vi "test_Timestamp Channel.vi"(8 "error in (no error)":errorcluster, 11 "TestCase in":refnum<class "Instrument Addon Common System Tests.lvclass">) -> (0 "error out":errorcluster, 3 "TestCase out":refnum<class "Instrument Addon Common System Tests.lvclass">)   [LabVIEW 2019, in "Instrument Addon Common System Tests.lvclass"]
uses:
  Instrument Addon Common System Tests.lvclass
  C:/Program Files (x86)/National Instruments/LabVIEW 2019/vi.lib/NI/VeriStand Custom Device Testing Tools/VeriStandTestCase/VeriStandTestCase.lvclass
  8f14a969-7c39-4f15-840b-a7ce507a422e.vi
  <vilib>/NI VeriStand/Execution/Workspace/NI VeriStand - Get Single Channel Value.vi
  <vilib>/NI VeriStand/Execution/Workspace/NI VeriStand - Set Single Channel Value.vi
  <vilib>/addons/_JKI Toolkits/VI Tester/TestCase.llb/TestCase.lvclass
  <vilib>/NI VeriStand/Execution/Workspace/NI_VS Workspace ExecutionAPI.lvlib
  C:/Program Files (x86)/National Instruments/LabVIEW 2019/vi.lib/addons/_JKI Toolkits/VI Tester/TestCase.llb/TestCase.lvclass
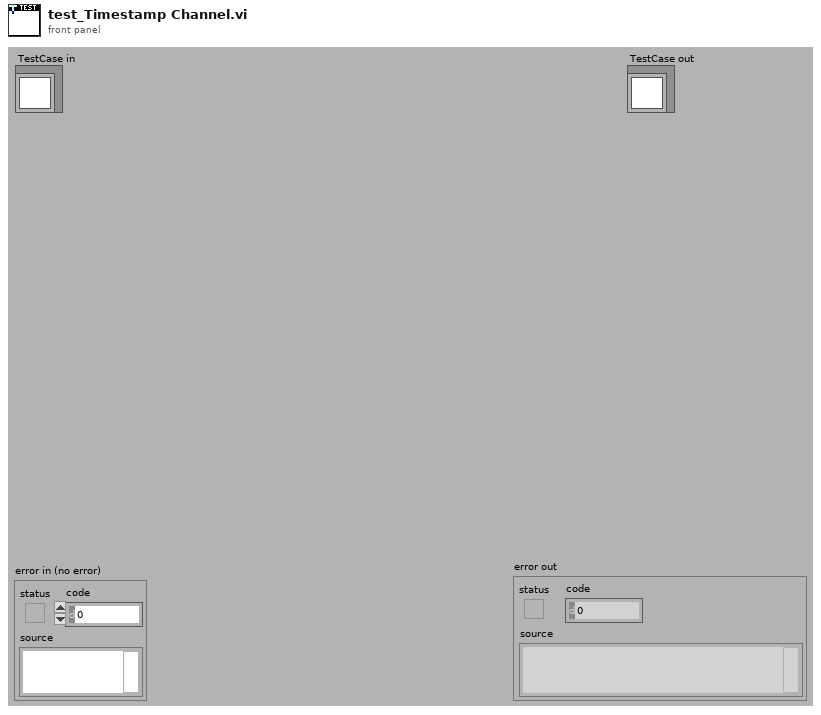
[diagram p1: front panel]
types:
  T1 = typedef "NI_VS Workspace ExecutionAPI.lvlib/WorkspaceAPI.ctl" = refnum<k24>
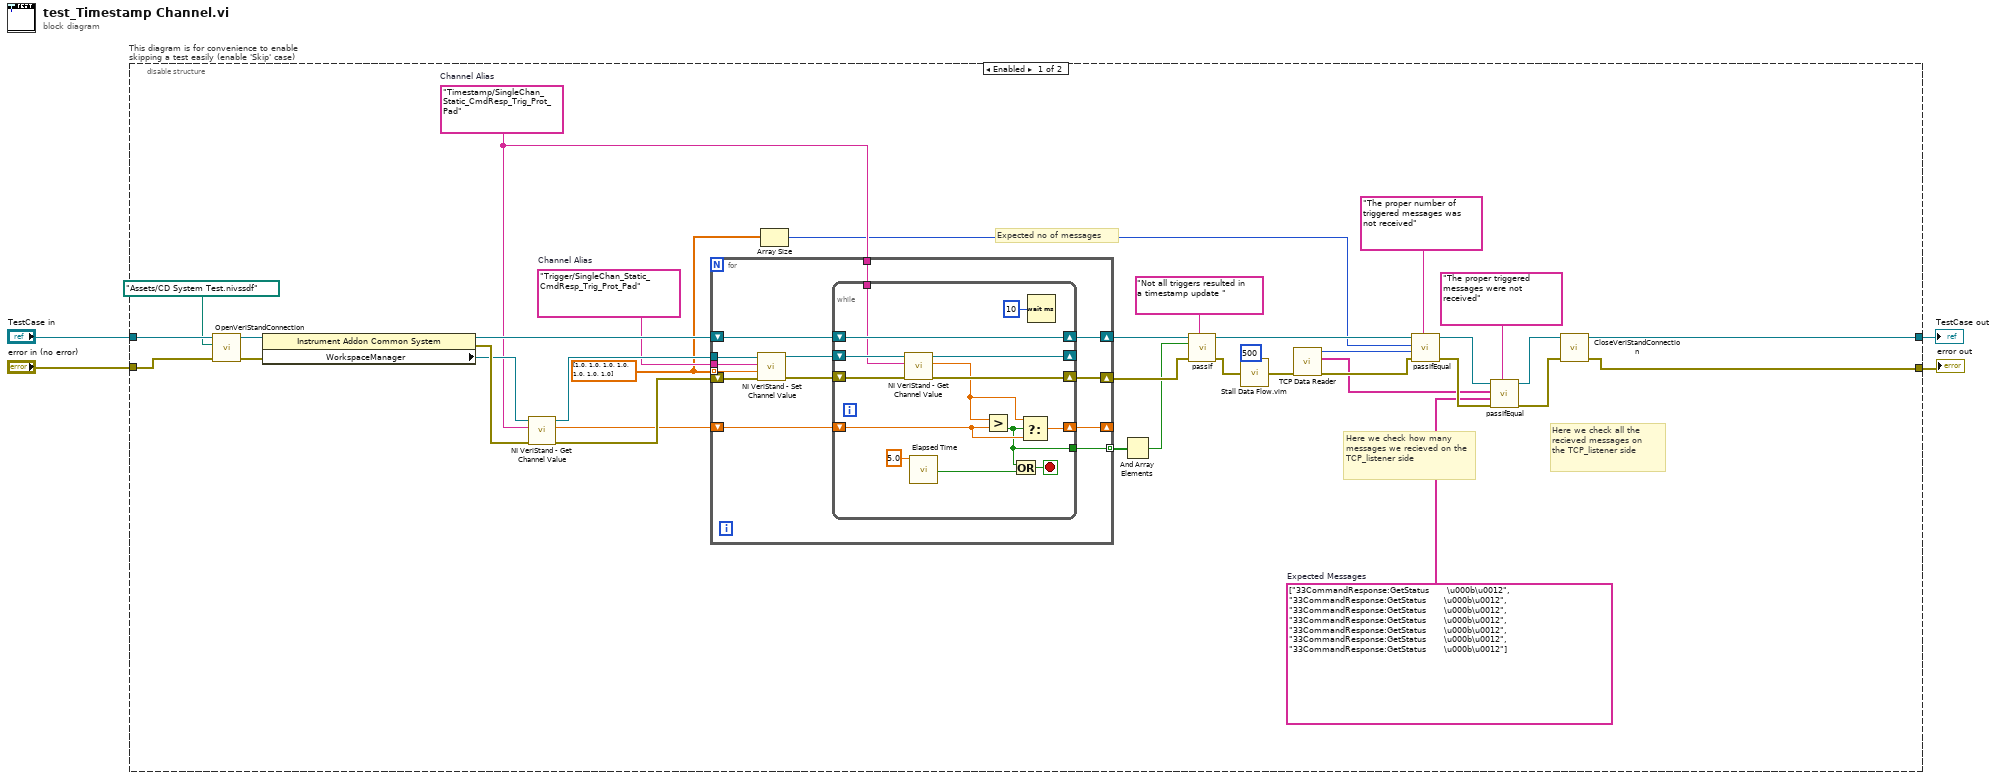
[diagram p0: block diagram]
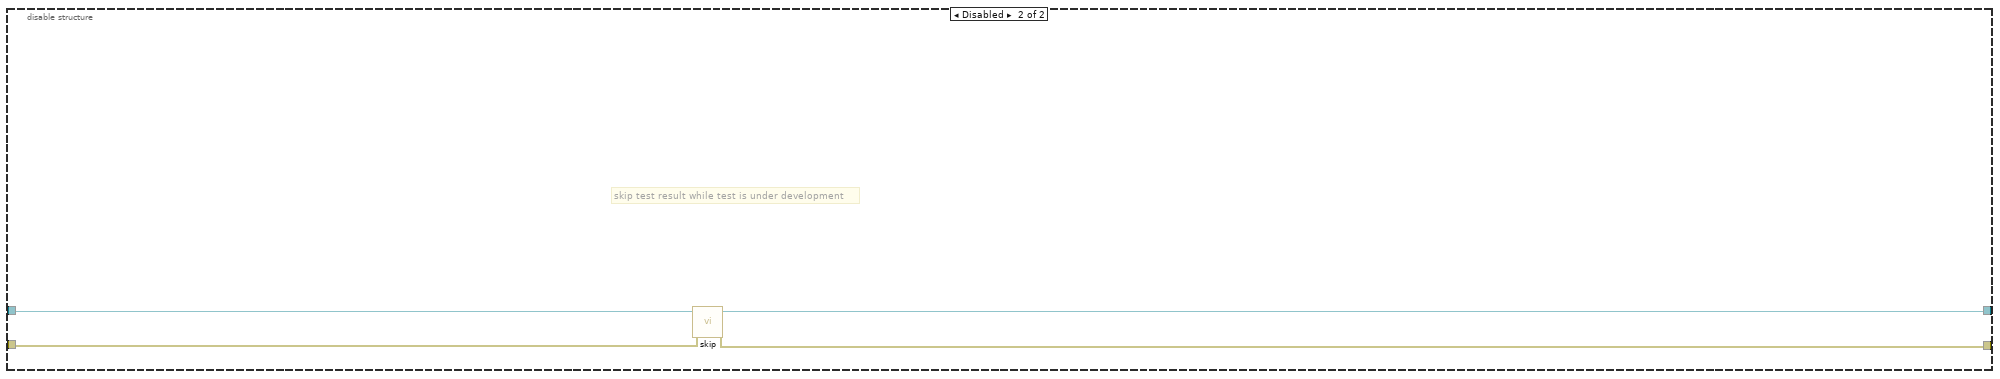
[diagram p2: hidden frame]
diagram:
  n1 = disable-structure "This diagram is for convenience to enable skipping a test easily (enable 'Skip' case)" shown="Enabled" {
    disable-tunnel: "TestCase in" -> [w38 w71]
    disable-tunnel: [w39 w69] -> w1
    disable-tunnel: [w40 w70] -> w3
    disable-tunnel: "error in (no error)" -> [w36 w68]
    frame Enabled {
      w11 = dbl[] [1.0, 1.0, 1.0, 1.0, 1.0, 1.0, 1.0]
      w18 = "Timestamp/SingleChan_Static_CmdResp_Trig_Prot_Pad"  # Channel Alias
      w28 = string[] ["33CommandResponse:GetStatus      \u000b\u0012", "33CommandResponse:GetStatus      \u000b\u0012", "33CommandResponse:GetStatus      \u000b\u0012", "33CommandResponse:GetStatus      \u000b\u0012", "33CommandResponse:GetStatus      \u000b\u0012", "33CommandResponse:GetStatus      \u000b\u0012", "33CommandResponse:GetStatus      \u000b\u0012"]  # Expected Messages
      w19 = "Trigger/SingleChan_Static_CmdResp_Trig_Prot_Pad"  # Channel Alias
      # "Expected no of messages"
      # "Here we check all the recieved messages on the TCP_listener side"
      # "Here we check how many messages we recieved on the TCP_listener side"
      n2 = call-dynamic "OpenVeriStandConnection.vi"("error in (no error)"=w36, "System Definition File"=path "Assets/CD System Test.nivssdf", "VeriStand Test Case in"=w38) -> ("error out"=w35:errorcluster, "VeriStand Test Case out"=w37:refnum<class "Instrument Addon Common System Tests.lvclass">)  [unwired: 6 in, 1 out]
      n3 = property class="Instrument Addon Common System "(reference=w37, error in=w35) -> (reference out=w33:refnum<class "Instrument Addon Common System Tests.lvclass">, error out=w24:errorcluster, "WorkspaceManager"=w23:T1)
      n4 = call-poly <vilib>:"NI VeriStand - Get Channel Value.vi"("error in (no error)"=w24, "Channel"=w18, "WorkspaceManager in"=w23) -> ("error out"=w22:errorcluster, "Value"=w20:dbl, "WorkspaceManager out"=w21:T1)  [unwired: 6 in]
      n5 = for {
        tunnel: w21 -> [w53]
        shift-right: [w45] -> w15
        shift-left: w22 -> [w52]
        shift-right: [w46] -> w16
        shift-left: w33 -> [w47]
        tunnel: w11 -> [w49] mode=indexing
        shift-right: [w44] -> _
        shift-left: w20 -> [w48]
        tunnel: w19 -> [w43]
        tunnel: w18 -> [w42]
        tunnel: [w41] -> w17 mode=indexing
        n6 = call-poly <vilib>:"NI VeriStand - Set Channel Value.vi"("error in (no error)"=w52, "Value"=w49, "Channel"=w43, "WorkspaceManager in"=w53) -> ("error out"=w50:errorcluster, "WorkspaceManager out"=w51:T1)  [unwired: 6 in]
        n7 = while {
          shift-right: [w65] -> _
          shift-left: w51 -> [w67]
          shift-right: [w64] -> w45
          shift-left: w50 -> [w66]
          shift-right: [w63] -> w46
          shift-left: w47 -> [w63]
          shift-right: [w62] -> w44
          shift-left: w48 -> [w56]
          tunnel: w42 -> [w61]
          tunnel: [w54] -> w41
          stop <- w59 stop-if-true
          n8 = call-poly <vilib>:"NI VeriStand - Get Channel Value.vi"("error in (no error)"=w66, "Channel"=w61, "WorkspaceManager in"=w67) -> ("error out"=w64:errorcluster, "Value"=w55:dbl, "WorkspaceManager out"=w65:T1)  [unwired: 6 in]
          n9 = call "Elapsed Time"("Time Target (s)"=5.0) -> ("Time has Elapsed"=w60:bool)  [unwired: 11 in, 7 out]
          n10 = Greater?(x=w55, y=w56) -> (0:w54:bool)
          n11 = Or(x=w54, y=w60) -> (x .or. y?=w59:bool)
          n12 = Select(t=w55, s=w54, f=w56) -> (s? t:f=w62:dbl)
          n13 = Wait (ms)(milliseconds to wait=u32 10) -> ()  [unwired: 1 out]
        }
      }
      n14 = Array Size(array=w11) -> (size(s)=w10:i32)
      n15 = And Array Elements(Boolean array=w17) -> (logical AND=w13:bool)
      n16 = call-dynamic "passIf.vi"("custom report message (\"\")"="Not all triggers resulted in a timestamp update " ("custom report message (\"\")"), "error in (no error)"=w15, "pass"=w13, "TestCase in"=w16) -> ("error out"=w7:errorcluster, "TestCase out"=w14:refnum<class "Instrument Addon Common System Tests.lvclass">)  [unwired: 6 in]
      n17 = call "Stall Data Flow.vim"("value in"=w7, "milliseconds to wait"=u32 500) -> ("value out"=w6:errorcluster)  [unwired: 1 out]
      n18 = call "TCP Data Reader.vi"("error in (no error)"=w6) -> ("error out"=w26:errorcluster, "Recieved Messages"=w25:string[], "No of messages"=w27:i32)  [unwired: 8 in]
      n19 = call-dynamic "passIfEqual.vi"("custom report message (\"\")"="The proper number of triggered messages was not received" ("custom report message (\"\")"), "error in (no error)"=w26, "y"=w27, "x"=w10, "TestCase in"=w14) -> ("error out"=w30:errorcluster, "TestCase out"=w32:refnum<class "Instrument Addon Common System Tests.lvclass">)  [unwired: 5 in]
      n20 = call-dynamic "passIfEqual.vi"("custom report message (\"\")"="The proper triggered messages were not received" ("custom report message (\"\")"), "error in (no error)"=w30, "y"=w28, "x"=w25, "TestCase in"=w32) -> ("error out"=w29:errorcluster, "TestCase out"=w31:refnum<class "Instrument Addon Common System Tests.lvclass">)  [unwired: 5 in]
      n21 = call-dynamic "CloseVeriStandConnection.vi"("error in (no error)"=w29, "VeriStand Test Case in"=w31) -> ("error out"=w40:errorcluster, "VeriStand Test Case out"=w39:refnum<class "Instrument Addon Common System Tests.lvclass">)  [unwired: 8 in]
    }
    frame Disabled {
      # "skip test result while test is under development"
      n22 = call <vilib>:"skip.vi"("error in (no error)"=w68, "TestCase in"=w71) -> ("error out"=w70:errorcluster, "TestCase out"=w69:refnum<class "Instrument Addon Common System Tests.lvclass">)  [unwired: 8 in]
    }
  }
  "error out" <- w3
  "TestCase out" <- w1
